vi "MAD_Header.vi"(8 "error in":errorcluster, 10 "HeaderArray":string[](array[string]), 11 "XLS in":refnum<class "XLS.lvclass">) -> (0 "error out":errorcluster, 3 "XLS out":refnum<class "XLS.lvclass">)   [LabVIEW 2017, in "Report_lib.lvlib" / "XLS.lvclass"]
doc: "This method performs and fullfill\ncommon Header for XLS report"
uses:
  XLS.lvclass
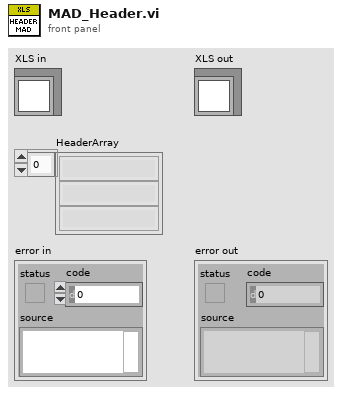
[diagram p1: front panel]
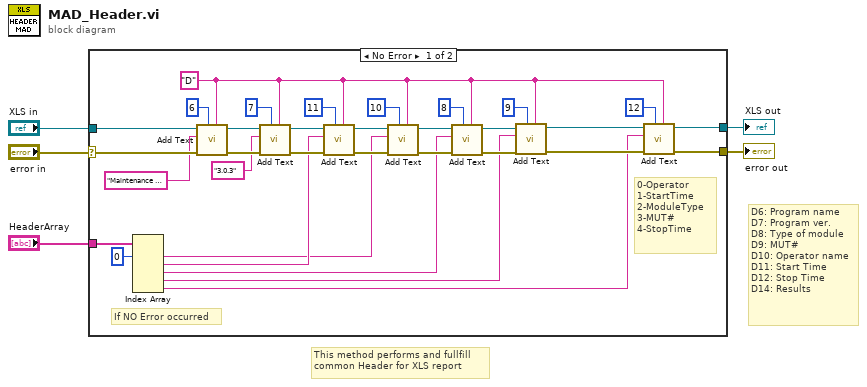
[diagram p0: block diagram]
diagram:
  # "This method performs and fullfill\ncommon Header for XLS report"
  # "D6: Program name\nD7: Program ver.\nD8: Type of module\nD9: MUT#\nD10: Operator name\nD11: Start Time\nD12: Stop Time\nD14: Results"
  n1 = case shown="No Error" "error in" {
    selector: "error in" -> [w38 w40]
    tunnel: [w12 w40] -> w4
    tunnel: [w13 w39] -> w2
    tunnel: "XLS in" -> [w37 w39]
    tunnel: "HeaderArray" -> [w28 _]
    frame No Error {
      w11 = "D" ("Adr")
      # "If NO Error occurred"
      # "0-Operator\n1-StartTime\n2-ModuleType\n3-MUT#\n4-StopTime"
      n2 = Index Array(array=w28, index #1=0 ("index")) -> (element #1=w23:string, element #2=w26:string, element #3=w18:string, element #4=w14:string, element #5=w6:string)  [unwired: 4 in]
      n3 = call "Add Text.vi"("Adr"=w11, "Index"=6, "error in"=w38, "text"="Maintenance & Diagnostic Cabinet", "XLS in"=w37) -> ("error out"=w34:errorcluster, "XLS out"=w35:refnum<class "XLS.lvclass">)  [unwired: 5 in]
      n4 = call "Add Text.vi"("Adr"=w11, "Index"=7, "error in"=w34, "text"="3.0.3", "XLS in"=w35) -> ("error out"=w30:errorcluster, "XLS out"=w31:refnum<class "XLS.lvclass">)  [unwired: 5 in]
      n5 = call "Add Text.vi"("Adr"=w11, "Index"=11, "error in"=w30, "text"=w26, "XLS in"=w31) -> ("error out"=w24:errorcluster, "XLS out"=w25:refnum<class "XLS.lvclass">)  [unwired: 5 in]
      n6 = call "Add Text.vi"("Adr"=w11, "Index"=10, "error in"=w24, "text"=w23, "XLS in"=w25) -> ("error out"=w20:errorcluster, "XLS out"=w21:refnum<class "XLS.lvclass">)  [unwired: 5 in]
      n7 = call "Add Text.vi"("Adr"=w11, "Index"=8, "error in"=w20, "text"=w18, "XLS in"=w21) -> ("error out"=w17:errorcluster, "XLS out"=w16:refnum<class "XLS.lvclass">)  [unwired: 5 in]
      n8 = call "Add Text.vi"("Adr"=w11, "Index"=9, "error in"=w17, "text"=w14, "XLS in"=w16) -> ("error out"=w7:errorcluster, "XLS out"=w8:refnum<class "XLS.lvclass">)  [unwired: 5 in]
      n9 = call "Add Text.vi"("Adr"=w11, "Index"=12, "error in"=w7, "text"=w6, "XLS in"=w8) -> ("error out"=w12:errorcluster, "XLS out"=w13:refnum<class "XLS.lvclass">)  [unwired: 5 in]
    }
    frame Error {
    }
  }
  "error out" <- w4
  "XLS out" <- w2
